vi "Get-all-properties-dialog.vi"(8 "error in (no error)":errorcluster, 11 "PF_MV1-D1312-240 in":refnum<class "PF_MV1-D1312-240.lvclass">) -> (0 "error out":errorcluster, 3 "PF_MV1-D1312-240 out":refnum<class "PF_MV1-D1312-240.lvclass">)   [LabVIEW 2013, in "CameraVision.lvlib" / "PF_MV1-D1312-240.lvclass"]
uses:
  PF_MV1-D1312-240.lvclass
  <userlib>/Photonfocus Toolkit/_Private/Controls/pf_Property_Cluster.ctl
  <userlib>/Photonfocus Toolkit/_Private/Controls/pf_Property_Type.ctl
  <userlib>/Photonfocus Toolkit/_Private/Controls/pf_Property_Flag.ctl
  Camera.lvclass/Camera.ctl
  Read IMAQ Session.vi
  <userlib>/Photonfocus Toolkit/Photonfocus_Toolkit.lvlib
panel:
  in  "OK":bool
  out "Properties Array":T1[](array[typedef])
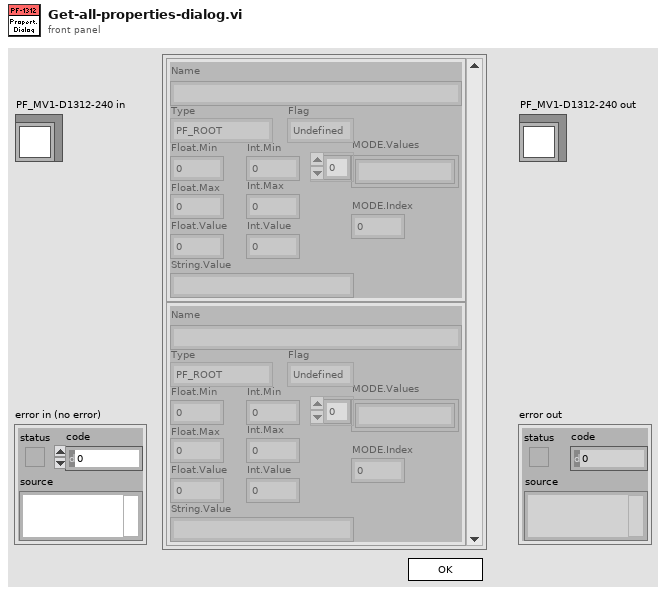
[diagram p1: front panel]
types:
  T1 = typedef "Photonfocus_Toolkit.lvlib/pf_Property_Cluster.ctl" = cluster{"Name":string, "Type":T2, "Float.Min":sgl, "Float.Max":sgl, "Float.Value":sgl, "Int.Min":u32, "Int.Max":u32, "Int.Value":u32, "String.Value":string, "MODE.Values":string[], "MODE.Index":i32, "Flag":T3}
  T2 = typedef "Photonfocus_Toolkit.lvlib/pf_Property_Type.ctl" = enum16{"Undefined", "PF_ROOT", "PF_INT", "PF_FLOAT", "PF_BOOL", "PF_MODE", "PF_REGISTER", "PF_STRING", "PF_BUFFER", "PF_STRUCT", "PF_ARRAY", "PF_COMMAND", "PF_EVENT"}
  T3 = typedef "Photonfocus_Toolkit.lvlib/pf_Property_Flag.ctl" = enum16{"Undefined", "RO", "WO", "RW"}
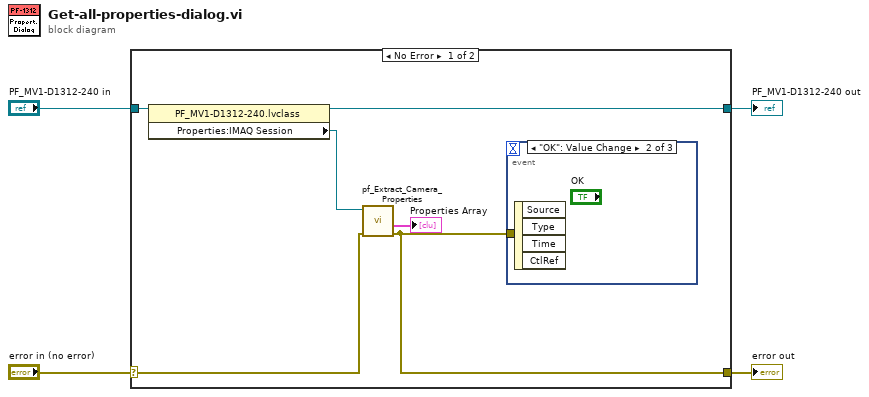
[diagram p0: block diagram]
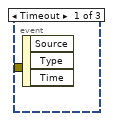
[diagram p2: hidden frame]
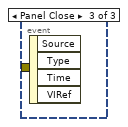
[diagram p3: hidden frame]
diagram:
  n1 = case shown="No Error" "error in (no error)" {
    selector: "error in (no error)" -> [w7 w12]
    tunnel: [w6 w12] -> w3
    tunnel: [w9 w11] -> w1
    tunnel: "PF_MV1-D1312-240 in" -> [w10 w11]
    frame No Error {
      n2 = property class="PF_MV1-D1312-240.lvclass"(reference=w10) -> (reference out=w9:refnum<class "PF_MV1-D1312-240.lvclass">, "Properties:IMAQ Session"=w8:refnum<k11>)  [unwired: 1 in, 1 out]
      n3 = call <userlib>:"pf_Extract_Camera_Properties.vi"("error in (no error)"=w7, "IMAQ Session in"=w8) -> ("error out"=w6:errorcluster, "Properties Array"=→"Properties Array":T1[])  [unwired: 8 out]
      n4 = event shown="[1] \"OK\": Value Change" {
        selector: _ -> [_ _ _]
        dyn-events: _ -> [_ _ _]
        timeout: _ -> [_ _ _]
        tunnel: w6 -> [_ _ _]
        event Timeout {
          n5 = event-data() -> ()  [unwired: 1 in, 3 out]
        }
        event "OK": Value Change {
          n6 = event-data() -> ()  [unwired: 1 in, 4 out]
        }
        event Panel Close {
          n7 = event-data() -> ()  [unwired: 1 in, 4 out]
        }
      }
    }
    frame Error {
    }
  }
  "error out" <- w3
  "PF_MV1-D1312-240 out" <- w1
